vi "loadXYpositions_svi.vi"(11 "Chemin en entrée":path) -> (2 "final XY":T1, 3 "Number of lines":u32)   [LabVIEW 2013]
uses:
  <vilib>/Analysis/Matrix/Datatypes/RealMatrix.ctl
  <vilib>/Analysis/Matrix/Numeric/Conversions/Array To Matrix - RA.vi
  <vilib>/Analysis/Matrix/NI_Matrix.lvlib
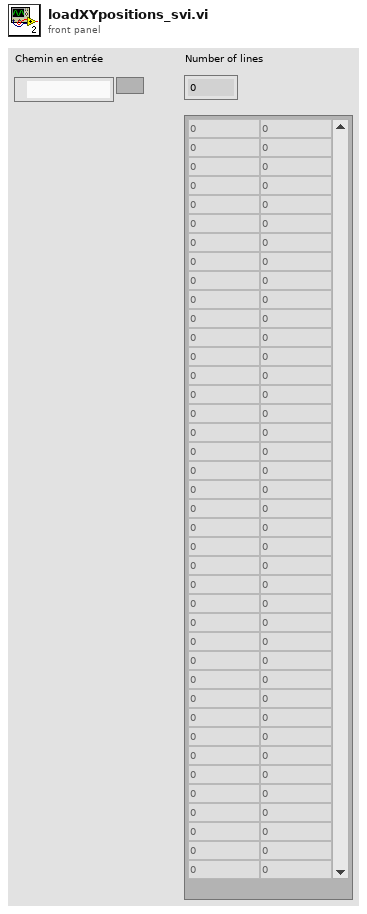
[diagram p1: front panel]
types:
  T1 = typedef "NI_Matrix.lvlib/RealMatrix.ctl" = dbl[][]
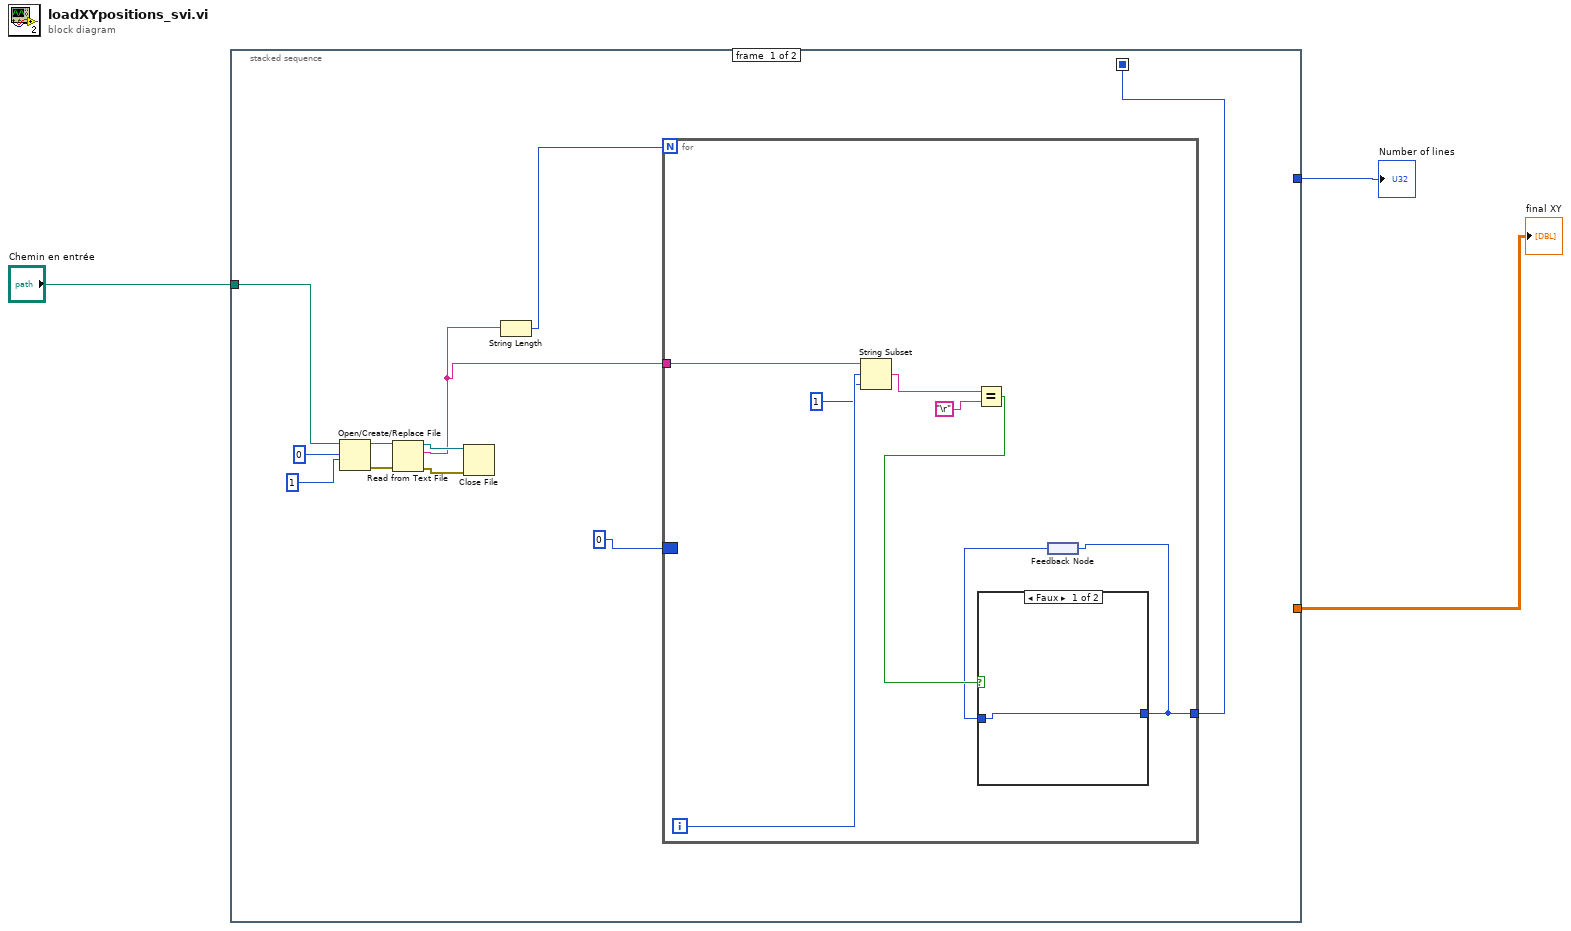
[diagram p0: block diagram]
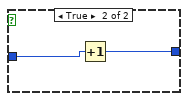
[diagram p2: hidden frame]
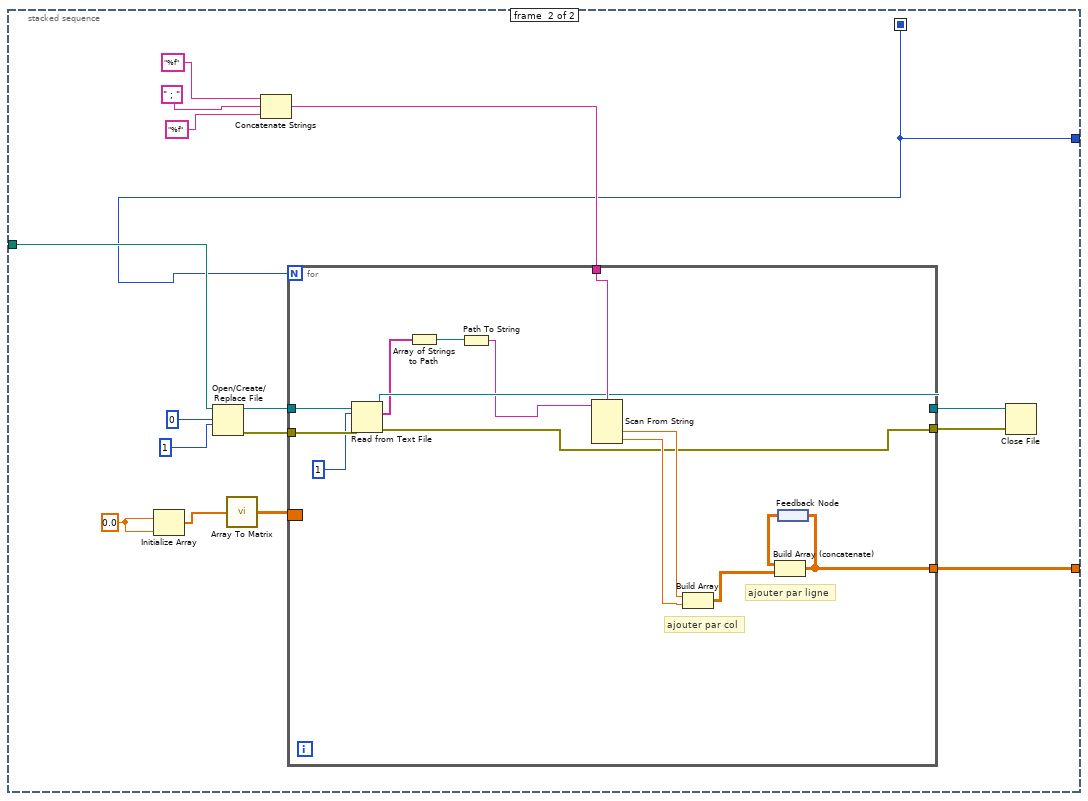
[diagram p3: hidden frame]
diagram:
  n1 = stacked-sequence {
    seq-local: [w4 _] -> [_ w26]
    tunnel: [_ w36] -> w1
    tunnel: "Chemin en entrée" -> [w12 w29]
    tunnel: [_ w26] -> w3
    frame #0 {
      n2 = Open/Create/Replace File(file path (use dialog)=w12, operation (0:open)=0, access (0:read/write)=1) -> (refnum out=w11:refnum<file>, error out=w10:errorcluster)  [unwired: 3 in, 1 out]
      n3 = Read from Text File(file (use dialog)=w11, error in=w10) -> (refnum out=w9:refnum<file>, text=w7:string, error out=w8:errorcluster)  [unwired: 2 in, 1 out]
      n4 = Close File(refnum=w9, error in=w8) -> ()  [unwired: 2 out]
      n5 = String Length(string=w7) -> (length=w6:i32)
      n6 = for {
        N: w6 -> [_]
        tunnel: w7 -> [w17]
        border: 0 -> [_]
        tunnel: [w15] -> w4
        i -> [w22]
        n7 = String Subset(string=w17, offset (0)=w22, length (rest)=1) -> (substring=w19:string)
        n8 = Equal?(x=w19, y="\r") -> (x = y?=w18:bool)
        n9 = feedback #1() -> (w16:i32)
        n10 = case shown="Faux" w18 {
          tunnel: [w23 w25] -> w15
          tunnel: w16 -> [w23 w24]
          frame False {
          }
          frame True {
            n11 = Increment(x=w24) -> (x+1=w25:i32)
          }
        }
        n12 = feedback-in #1(w15) -> ()
      }
    }
    frame #1 {
      w38 = 0.0
      n13 = Initialize Array(w38, w38) -> (w39:dbl[])
      n14 = Open/Create/Replace File(file path (use dialog)=w29, operation (0:open)=0, access (0:read/write)=1) -> (refnum out=w30:refnum<file>, error out=w41:errorcluster)  [unwired: 3 in, 1 out]
      n15 = call-poly <vilib>:"Array To Matrix.vi"("Real 1D Array"=w39) -> ("Real Matrix (Column Vector)"=w37:T1)
      n16 = Concatenate Strings("%f" ("chaîne"), " ; ", "%f" ("chaîne")) -> (w31:string)
      n17 = for {
        N: w26 -> [_]
        tunnel: w30 -> [w52]
        tunnel: w41 -> [w51]
        tunnel: [w45] -> w28
        tunnel: [w46] -> w27
        border: w37 -> [_]
        tunnel: [w53] -> w36
        tunnel: w31 -> [w49]
        # "ajouter par ligne"
        # "ajouter par col"
        n18 = Read from Text File(file (use dialog)=w52, count=1, error in=w51) -> (refnum out=w45:refnum<file>, text=w43:string[], error out=w46:errorcluster)  [unwired: 1 in, 1 out]
        n19 = Array of Strings to Path(0:w43) -> (2:w44:path)  [unwired: 1 in]
        n20 = Path To String(path=w44) -> (string=w42:string)
        n21 = Scan From String(format string=w49, input string=w42) -> (output 1=w47:dbl, output 2=w48:dbl)  [unwired: 4 in, 3 out]
        n22 = Build Array(w47, w48) -> (w55:T1)
        n23 = feedback #2() -> (w54:T1)
        n24 = Build Array (concatenate)(w54, w55) -> (w53:T1)
        n25 = feedback-in #2(w53) -> ()
      }
      n26 = Close File(refnum=w28, error in=w27) -> ()  [unwired: 2 out]
    }
  }
  "final XY" <- w1
  "Number of lines" <- w3
